vi "NoLogTypeDefined--error.vi"() -> (0 "Error Out":errorcluster)   [LabVIEW 2019, in "TSC Event Logger.lvlib"]
doc: "No log type defined error. \n\nCode: -8000\n\n<b>Code Developed By:</b>\nTechnology Service Corporation\nBloomington, IN 47403\nwww.tsc.com/atcs\n\nDeveloper:\nDaniel Coons"
uses:
  TSC Event Logger.lvlib
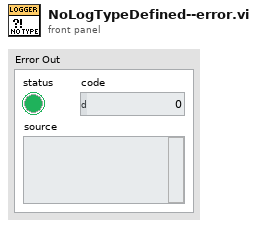
[diagram p1: front panel]
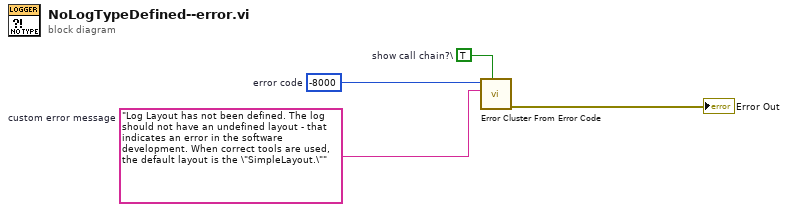
[diagram p0: block diagram]
diagram:
  w4 = -8000  # error code
  w3 = "Log Layout has not been defined. The log should not have an undefined layout - that indicates an error in the software development. When correct tools are used, the default layout is the \"SimpleLayout.\""  # custom error message
  w2 = TRUE  # show call chain?\
  n1 = call <vilib>:"Error Cluster From Error Code.vi"("show call chain? (False)"=w2, "error message (\"\")"=w3, "error code (0)"=w4) -> ("error out"=→"Error Out":errorcluster)  [unwired: 6 in]
